vi "Test Start Window Drag.vi"() -> ()   [LabVIEW 2021]
panel:
  in  "stop":bool
  out "Boolean":bool
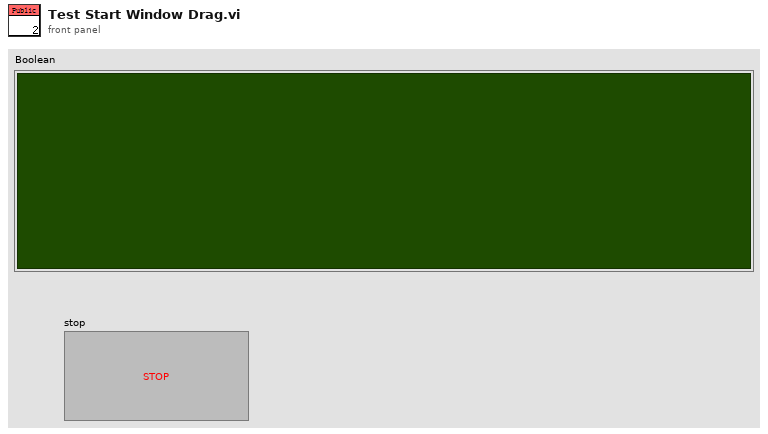
[diagram p1: front panel]
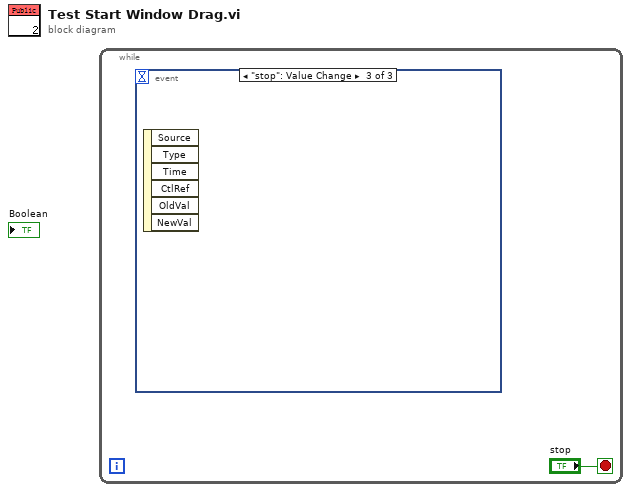
[diagram p0: block diagram]
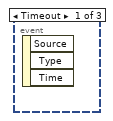
[diagram p2: hidden frame]
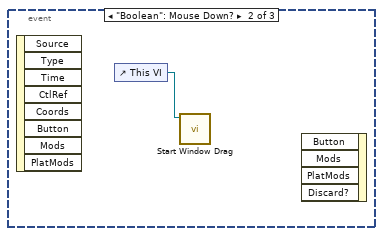
[diagram p3: hidden frame]
diagram:
  n1 = while {
    stop <- "stop" stop-if-true
    n2 = event shown="[2] \"stop\": Value Change" {
      selector: _ -> [_ _ _]
      dyn-events: _ -> [_ _ _]
      timeout: _ -> [_ _ _]
      event Timeout {
        n3 = event-data() -> ()  [unwired: 1 in, 3 out]
      }
      event "Boolean": Mouse Down? {
        n4 = event-data() -> ()  [unwired: 1 in, 8 out]
        n5 = control-ref of="This VI"() -> (w2:refnum<vi>)
        n6 = call "Start Window Drag.vi"("VI Ref (calling VI)"=w2) -> ()  [unwired: 9 in, 2 out]
        n7 = event-data() -> ()  [unwired: 5 in, 1 out]
      }
      event "stop": Value Change {
        n8 = event-data() -> ()  [unwired: 1 in, 6 out]
      }
    }
  }
